vi "Auto Number Get Next SSN.vi"(8 "error in (no error)":errorcluster, 9 "Initial Serial Number (1)":string, 10 "Model Number":string, 11 "Connection Refnum":T1) -> (0 "error out":errorcluster, 1 "Current Number":i32, 2 "Spartan Serial Number":string, 3 "Connection Refnum":T1)   [LabVIEW 2011]
uses:
  Summitek EXT/ODBC/SQL Controls/Connection Refnum.ctl
  Auto Number Record.ctl
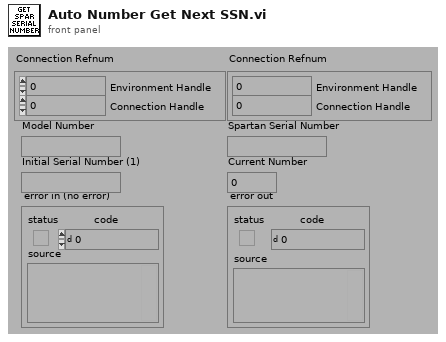
[diagram p1: front panel]
types:
  T1 = typedef "Connection Refnum.ctl" = cluster{"Environment Handle":i32, "Connection Handle":i32}
  T2 = typedef "Auto Number Record.ctl" = cluster{"ixAutoNumber":i32, "sModelNumber":string, "sSerialNumber":string}
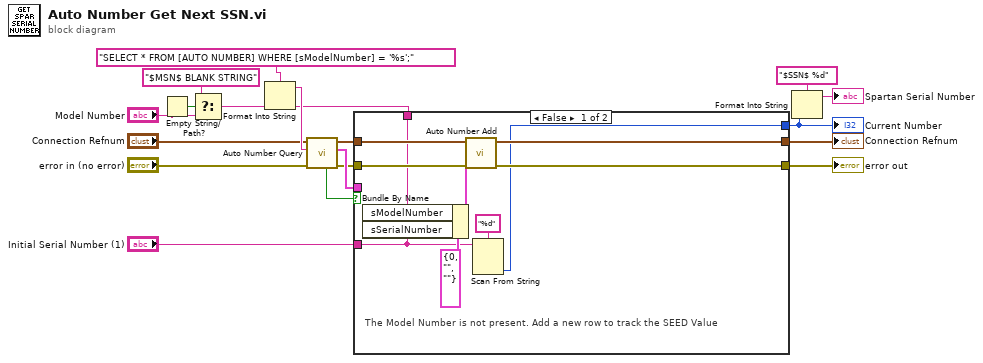
[diagram p0: block diagram]
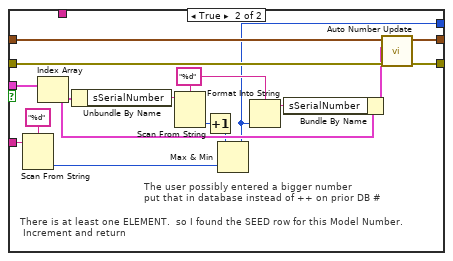
[diagram p2: hidden frame]
diagram:
  n1 = Empty String/Path?(string/path="Model Number") -> (empty?=w10:bool)
  n2 = Select(t="$MSN$ BLANK STRING", s=w10, f="Model Number") -> (s? t:f=w7:string)
  n3 = Format Into String(format string="SELECT * FROM [AUTO NUMBER] WHERE [sModelNumber] = '%s';" ("Query"), w7) -> (resulting string=w18:string)  [unwired: 2 in, 1 out]
  n4 = call "Auto Number Query.vi"("error in (no error)"="error in (no error)", "Query"=w18, "Connection Refnum"="Connection Refnum") -> ("error out"=w14:errorcluster, "Auto Number Records"=w16:T2[], "Connection Refnum"=w15:T1, "Data Present?"=w17:bool)  [unwired: 5 out]
  n5 = case shown="False" w17 {
    tunnel: w16 -> [_ w44]
    tunnel: w15 -> [w26 w42]
    tunnel: w14 -> [w25 w41]
    tunnel: [w27 w40] -> w3
    tunnel: [w28 w39] -> w4
    tunnel: [w20 w31] -> w6
    tunnel: w7 -> [w22 _]
    tunnel: "Initial Serial Number (1)" -> [w19 w35]
    frame False {
      # "The Model Number is not present. Add a new row to track the SEED Value"
      n6 = Bundle By Name(cluster=T2 {"ixAutoNumber"=0, "sModelNumber"="", "sSerialNumber"=""} ("Auto_Number Record"), "sModelNumber"=w22, "sSerialNumber"=w19) -> (w23:T2)
      n7 = call "Auto Number Add.vi"("error in (no error)"=w25, "Auto Number Record"=w23, "Connection Refnum"=w26) -> ("error out"=w27:errorcluster, "Connection Refnum"=w28:T1)  [unwired: 7 out]
      n8 = Scan From String(format string="%d", input string=w19) -> (output 1=w20:i32)  [unwired: 2 in, 4 out]
    }
    frame True {
      w36 = "%d" ("format string")
      # "The user possibly entered a bigger number\nput that in database instead of ++ on prior DB #"
      # "There is at least one ELEMENT.  so I found the SEED row for this Model Number.\n Increment and return"
      n9 = Scan From String(format string="%d", input string=w35) -> (output 1=w32:i32)  [unwired: 2 in, 4 out]
      n10 = Index Array(array=w44) -> (element=w38:T2)  [unwired: 1 in]
      n11 = Unbundle By Name(w38) -> ("sSerialNumber"=w29:string)
      n12 = Scan From String(format string=w36, input string=w29) -> (output 1=w43:i32)  [unwired: 2 in, 4 out]
      n13 = Increment(x=w43) -> (x+1=w33:i32)
      n14 = Max & Min(x=w33, y=w32) -> (max(x,y)=w31:i32)  [unwired: 1 out]
      n15 = Format Into String(format string=w36, w31) -> (resulting string=w30:string)  [unwired: 2 in, 1 out]
      n16 = Bundle By Name(cluster=w38, "sSerialNumber"=w30) -> (w37:T2)
      n17 = call "Auto Number Update.vi"("error in (no error)"=w41, "Auto Number Record"=w37, "Connection Refnum"=w42) -> ("error out"=w40:errorcluster, "Connection Refnum"=w39:T1)  [unwired: 7 out]
    }
  }
  "error out" <- w3
  "Current Number" <- w6
  "Connection Refnum" <- w4
  n18 = Format Into String(format string="$SSN$ %d", w6) -> (resulting string=→"Spartan Serial Number":string)  [unwired: 2 in, 1 out]
